vi "OnDataChange.vi"(0 "StepMotorController in":refnum<class "StepMotorController.lvclass">, 1 "DataExchange":T1, 3 "error in (no error)":errorcluster) -> (7 "StepMotorController out":refnum<class "StepMotorController.lvclass">, 10 "error out":errorcluster)   [LabVIEW 2020]
uses:
  StepMotorController.lvclass
  Model/Hardware Abstraction Layer/Component/Device/Device/DataExchange.ctl
  Interface/DataListener/DataListener.lvclass
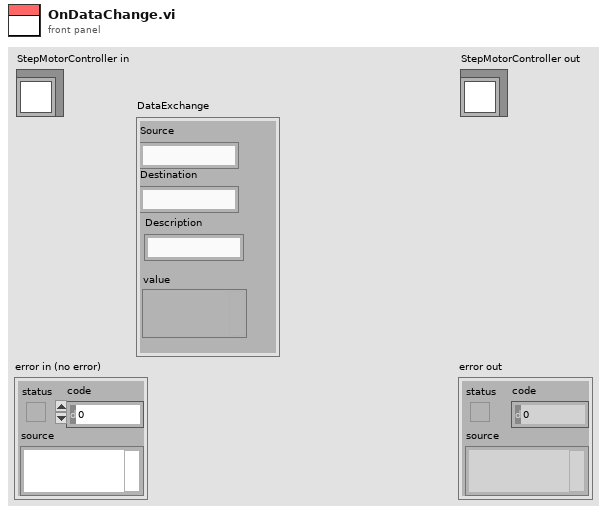
[diagram p1: front panel]
types:
  T1 = typedef "DataListener.lvclass/DataExchange.ctl" = cluster{"Source":string, "Destination":string, "Description":string, "value":variant}
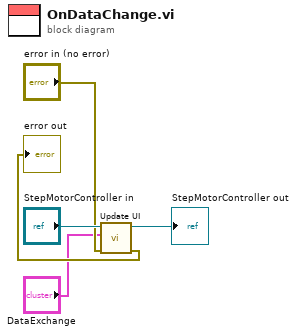
[diagram p0: block diagram]
diagram:
  n1 = call-dynamic "Update UI.vi"("error in (no error)"="error in (no error)", "DataExchange"="DataExchange", "StepMotorController in"="StepMotorController in") -> ("error out"=→"error out":errorcluster, "StepMotorController out"=→"StepMotorController out":refnum<class "StepMotorController.lvclass">)  [unwired: 7 in]
